vi "Current Write Array.vi"(8 "error in":errorcluster, 10 "Current.AV":dbl[](array[numeric]), 11 "Device in":refnum<class "Device.lvclass">) -> (0 "error out":errorcluster, 3 "Device out":refnum<class "Device.lvclass">)   [LabVIEW 2023, in "Device.lvclass"]
uses:
  Device.lvclass
  Low Level Capabilities/Current/Current Actual Value/Current Actual Value.lvclass
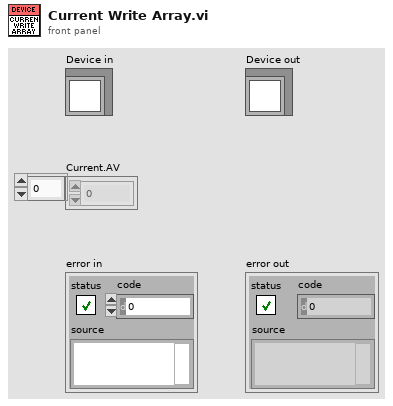
[diagram p1: front panel]
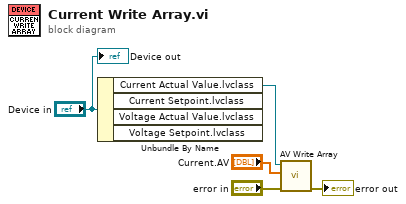
[diagram p0: block diagram]
diagram:
  n1 = Unbundle By Name("Device in") -> ("Current Actual Value.lvclass"=w4:refnum<class "Current Actual Value.lvclass">)  [unwired: 3 out]
  n2 = call-dynamic "AV Write Array.vi"("error in"="error in", "Current AV"="Current.AV", "Current Actual Value in"=w4) -> ("error out"=→"error out":errorcluster)  [unwired: 7 in, 1 out]
  "Device out" <- "Device in"
